vi "FPGA myRIOMain_v10.vi"() -> ()   [LabVIEW 2019]
doc: "Main FPGA VI\nUse the bitfile generated by this VI in the real-time code.\n\nv5: 16-pt Moving Average filter in AI sample loop"
uses:
  TypeDefs/AO mode TabCtrl.ctl
  TypeDefs/SamplingModeEnum_v2.ctl
  <vilib>/Platform/TimedLoop/XDataNode/timing_clust.ctl
  <vilib>/Platform/TimedLoop/XDataNode/nitl_modes.ctl
  <vilib>/Platform/TimedLoop/XDataNode/wakeup.ctl
  <vilib>/rvi/Emulation/niFpgaGetClockAttributes.vi
  <vilib>/rvi/Emulation/niFpgaSctlEmulationGetInTimedLoop.vi
  <vilib>/rvi/Emulation/niFpgaEmulationReportErrorSimple.vi
  <vilib>/rvi/eio/common/nirviEmuTemplateMethod_errors.vi
  <vilib>/rvi/Emulation/niFpgaEmulationIsFPGAContextNoSignature.vi
  <vilib>/rvi/errors/niFpgaSetErrorForExecOnDevCompSimple.vi
  <vilib>/rvi/eio/common/nirviEmuReportErrorAndStop.vi
  <vilib>/rvi/DataTransferAndStorage/Container/Common/niFpgaContainerGetUniqueNameForEmu.vi
  <vilib>/rvi/FIFO/Fifo_Resource/nirvififoEmulationSetSize.vi
  <vilib>/rvi/FIFO/Fifo_Resource/nirviFifoEmulationQueueMgr.vi
  <instcachedir>/0/nirviFifoEmulationQueueMgr_E5CAEC123FF24DC58D834DCA3CDAA9B5.lvgen/nirviFifoEmulationQueueMgr_E5CAEC123FF24DC58D834DCA3CDAA9B5_003.vi
  <vilib>/rvi/FIFO/Fifo_Resource/nirvififoEmulationDetermineInputValidOut.vi
  <vilib>/rvi/FIFO/Fifo_Resource/nirvififoEmulationCreateLock.vi
  <vilib>/rvi/Emulation/niFpgaProcessEmulError.vi
  <vilib>/rvi/FIFO/Fifo_Resource/nirvififoEmulationObtainLock.vi
  <vilib>/rvi/FIFO/Fifo_Resource/nirvififoEmulationReleaseLock.vi
  <vilib>/rvi/occurrence/nirviWaitOnOccurrenceBase.vi
  <vilib>/rvi/errors/nirviReportUnexpectedCaseInternalError.vi
  <vilib>/rvi/errors/nirviReportUnexpectedCaseInternalError (U32).vi
  <vilib>/rvi/Emulation/niFpgaCriticalErrorInLSC.vi
  <vilib>/Utility/error.llb/Clear Errors.vi
  <vilib>/rvi/Analysis/common/codeGenErrors/XNode/niFpgaXNodeCodeGenErrorHandle.vi
  <vilib>/eio/EIONode/EIONode.xnode
  <vilib>/rvi/DataTransferAndStorage/Container/XNode/niFpgaContainer.xnode
  <vilib>/rvi/FIFO/Fifo_Resource/nirvififoEmulationWrite.vi
  <vilib>/rvi/FIFO/Fifo_Resource/nirvififoEmulationRead.vi
  <vilib>/rvi/Analysis/measure/butterworth/XNode/niFpgaButterworthFilter.xnode
  <vilib>/rvi/FXPMathLib/FxpMul/XNode/nifxpmath_Multiplier.xnode
  <vilib>/rvi/Analysis/measure/LMRsmpl/XNode/niFPGA Rational Resampler.xnode
  <vilib>/Platform/TimedLoop/XDataNode/XDataNode.xnode
  FPGA functions/FPGA functions.lvlib
  <vilib>/Platform/TimedLoop/XDataNode/XDNodeRunTimeDep.lvlib
  <vilib>/rvi/FXPMathLib/sim/FxpSim.dll
panel:
  in  "scaled BW coefficients":i32[](array[numeric])=[-850883994, 1909449570, 3794062, -975456236, 2033039520, 4039635]
  in  "Sampling Mode":T1
  in  "AI Proc. Count [ticks]":u32
  in  "AI Count [ticks]":u32
  out "AI M Loop time [ticks]":u32
  out "FPGA AI DMA\nOverflow?":bool
  out "Sample Freq. \ntoo high?":bool
  out "Processing Loop time [ticks]":u32
  in  "AO mode":T2
  in  "AO Out [V]":fxp<+/-,18,5> format="%#.6g"
  in  "AO enable?":bool
  out "AI In [V]":fxp<+/-,24,5> format="%#.10g"
  out "FPGA AO DMA\nOverflow?":bool
  out "Int. Output":i16
  out "Raw Int. Input":fxp<+/-,22,12> format="%.8g"
  out "AO Loop time [ticks]":u32
  out "AI Loop time [ticks]":u32
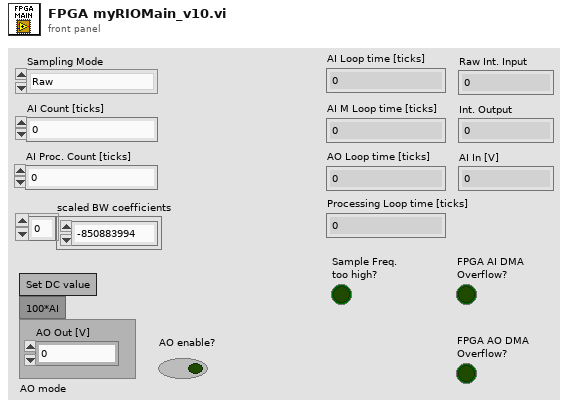
[diagram p1: front panel]
types:
  T1 = typedef "SamplingModeEnum_v2.ctl" = enum16{"Raw", "M64 - Resampling", "2nd-order Butterworth", "4th-order Butterworth", "64pt-MA", "128pt-MA", "256pt-MA"}
  T2 = typedef "AO mode TabCtrl.ctl" = enum32{"Set DC value", "100*AI"}
  T3 = typedef "XDNodeRunTimeDep.lvlib/timing_clust.ctl" = cluster{"Expected End [f-1]":u64, "Actual End [f-1]":u64, "Finished Late? [f-1]":bool, "Expected End [i-1]":u64, "Actual End [i-1]":u64, "Finished Late? [i-1]":bool, "Expected Start [i]":u64, "Actual Start [i]":u64, "Expected Start [f]":u64, "Actual Start [f]":u64, "Source Name":string, "Structure Name":string, "Period":i64, "Deadline":i64, "Offset":i64, "Start":i64, "Priority":i32, "Timeout":i32, "Mode":T4, "Wakeup Reason":T5, "Error":errorcluster, "Source Type":string, "Secondary Source Type":string, "Global End Time":u64, "Global Start Time":u64, "Frame Duration":u64, "Iteration Duration":u64, "Assigned CPU":i32, "I/O Scan Engine Mode":u32}
  T4 = typedef "XDNodeRunTimeDep.lvlib/nitl_modes.ctl" = enum32{"No Change", "Process missed periods, maintain original phase", "Discard missed periods, maintain original phase", "Process missed periods, ignore original phase", "Discard missed periods, ignore original phase"}
  T5 = typedef "XDNodeRunTimeDep.lvlib/wakeup.ctl" = enum32{"Normal", "Aborted", "Asynchronous wakeup", "Timing source error", "Timed loop error", "Timeout"}
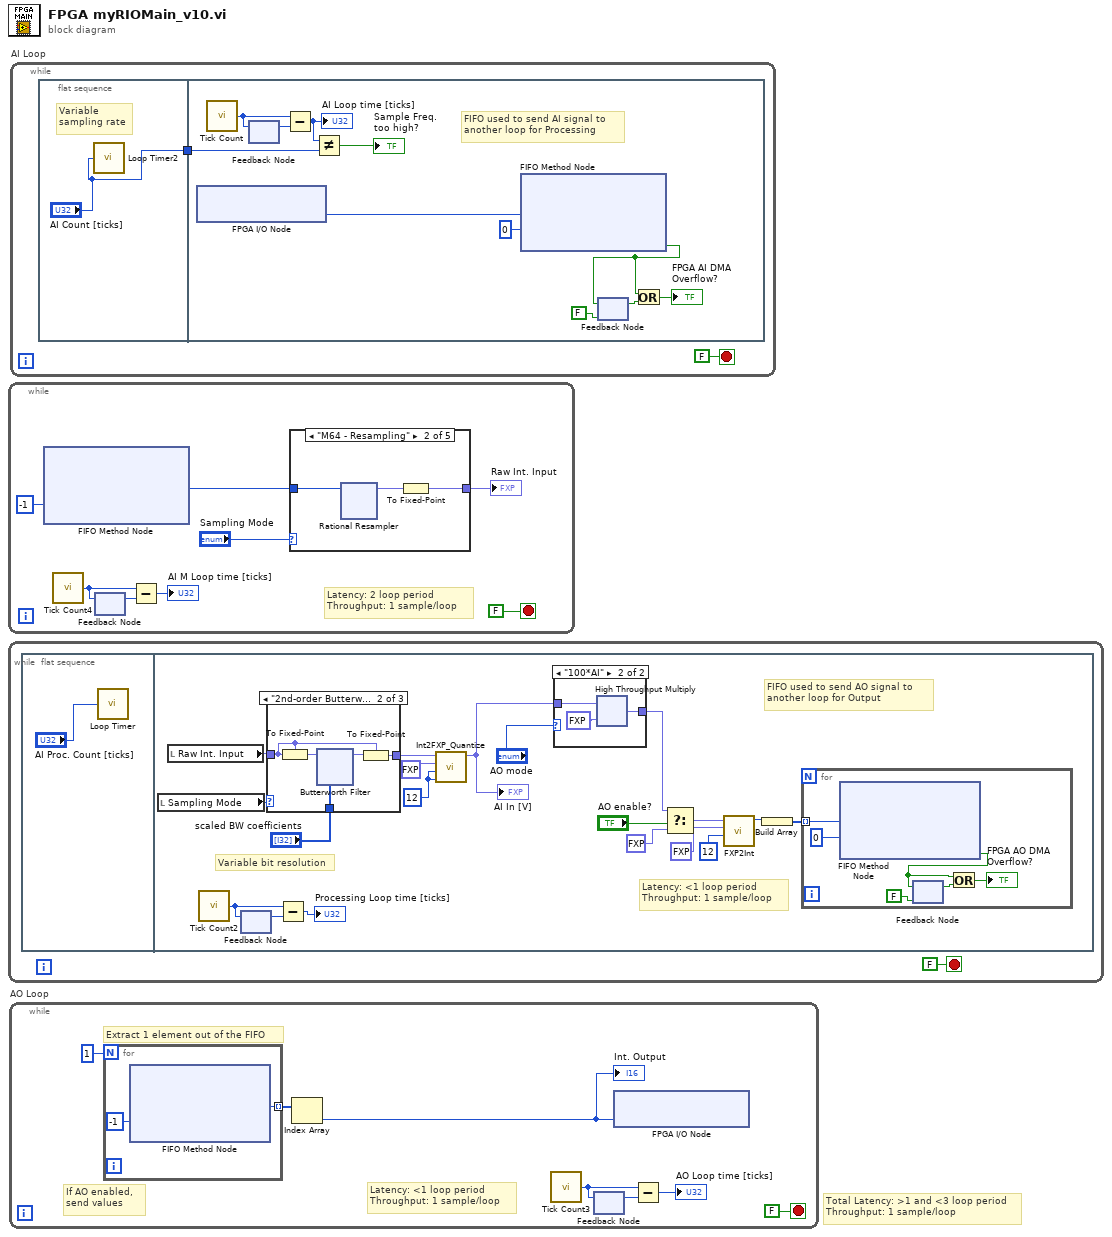
[diagram p0: block diagram]
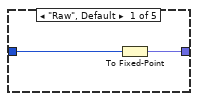
[diagram p2: hidden frame]
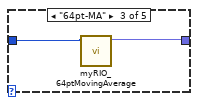
[diagram p3: hidden frame]
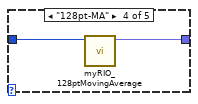
[diagram p4: hidden frame]
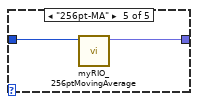
[diagram p5: hidden frame]
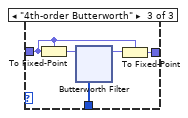
[diagram p7: hidden frame]
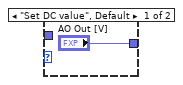
[diagram p8: hidden frame]
diagram:
  # "Total Latency: >1 and <3 loop period\nThroughput: 1 sample/loop"
  n1 = while {
    stop <- FALSE stop-if-true
    # "Latency: 2 loop period\nThroughput: 1 sample/loop"
    n2 = xnode ("FIFO Method Node")("Timeout"=-1) -> ("Element"=w1:i16)  [unwired: 1 in, 2 out]
    n3 = call "Tick Count4"() -> ("Tick Count(Ticks)"=w7:u32)
    n4 = feedback #1() -> (w6:u32)  [unwired: 1 in]
    n5 = feedback-in #1(w7) -> ()
    n6 = Subtract(x=w7, y=w6) -> (x-y=→"AI M Loop time [ticks]":u32)
    n7 = case shown="\"M64 - Resampling\"" "Sampling Mode" {
      tunnel: [w10 w11 w48 w50 w52] -> w3
      tunnel: w1 -> [w9 w13 w49 w51 w53]
      frame "Raw", Default {
        n8 = To Fixed-Point(number=w9) -> (fixed-point=w10:fxp<+/-,22,12>)  [unwired: 1 in]
      }
      frame "M64 - Resampling" {
        n9 = xnode "Rational Resampler"("input data"=w13) -> ("output data"=w12:fxp<+/-,18,16>)  [unwired: 2 out]
        n10 = To Fixed-Point(number=w12) -> (fixed-point=w11:fxp<+/-,22,12>)  [unwired: 1 in]
      }
      frame "64pt-MA" {
        n11 = call "myRIO_64ptMovingAverage.vi"("Raw input"=w49) -> ("Avg. output"=w48:fxp<+/-,22,12>)  [unwired: 10 in]
      }
      frame "128pt-MA" {
        n12 = call "myRIO_128ptMovingAverage.vi"("Raw input"=w51) -> ("Avg. output"=w50:fxp<+/-,22,12>)  [unwired: 10 in]
      }
      frame "256pt-MA" {
        n13 = call "myRIO_256ptMovingAverage.vi"("Raw input"=w53) -> ("Avg. output"=w52:fxp<+/-,22,12>)  [unwired: 10 in]
      }
    }
    "Raw Int. Input" <- w3
  }
  n14 = while {
    stop <- FALSE stop-if-true
    n15 = flat-sequence {
      frame #0 {
        n16 = call "Loop Timer"("Count(Ticks)"="AI Proc. Count [ticks]") -> ()  [unwired: 1 out]
      }
      frame #1 {
        w56 = i8 12 ("Input Bit resolution")
        # "Variable bit resolution"
        # "Latency: <1 loop period\nThroughput: 1 sample/loop"
        # "FIFO used to send AO signal to \nanother loop for Output"
        n17 = local read "Sampling Mode"() -> (w61:T1)
        n18 = local read "Raw Int. Input"() -> (w62:fxp<+/-,22,12>)
        n19 = call "Tick Count2"() -> ("Tick Count(Ticks)"=w65:u32)
        n20 = feedback #2() -> (w64:u32)  [unwired: 1 in]
        n21 = feedback-in #2(w65) -> ()
        n22 = case shown="\"2nd-order Butterworth\"" w61 {
          tunnel: [w75 w79 w92] -> w59
          tunnel: w62 -> [w75 w76 w89]
          tunnel: "scaled BW coefficients" -> [_ w77 w90]
          frame "Raw", Default {
          }
          frame "2nd-order Butterworth" {
            n23 = To Fixed-Point(fixed-point type=w76, number=w76) -> (fixed-point=w80:fxp<+/-,22,12>)
            n24 = xnode "Butterworth Filter"("input data"=w80, "scaled coefficients"=w77) -> ("output data"=w78:fxp<+/-,26,16>)  [unwired: 1 in]
            n25 = To Fixed-Point(fixed-point type=w76, number=w78) -> (fixed-point=w79:fxp<+/-,22,12>)
          }
          frame "4th-order Butterworth" {
            n26 = To Fixed-Point(fixed-point type=w89, number=w89) -> (fixed-point=w93:fxp<+/-,22,12>)
            n27 = xnode "Butterworth Filter"("input data"=w93, "scaled coefficients"=w90) -> ("output data"=w91:fxp<+/-,26,16>)  [unwired: 1 in]
            n28 = To Fixed-Point(fixed-point type=w89, number=w91) -> (fixed-point=w92:fxp<+/-,22,12>)
          }
        }
        n29 = Subtract(x=w65, y=w64) -> (x-y=→"Processing Loop time [ticks]":u32)
        n30 = call "Int2FXP_Quantize.vi"("Output Bit resolution"=w56, "Input Bit resolution"=w56, "Multiplier"=fxp<+,8,4> 10.0, "Input (Int)"=w59) -> ("Output (FXP)"=w58:fxp<+/-,24,5>)  [unwired: 7 in]
        "AI In [V]" <- w58
        n31 = case shown="\"100*AI\"" "AO mode" {
          tunnel: ["AO Out [V]" w103] -> w67
          tunnel: w58 -> [_ w105]
          frame "Set DC value", Default {
          }
          frame "100*AI" {
            n32 = xnode ("High Throughput Multiply")("x"=w105, "y"=fxp<+,5,7> 100.0) -> ("x*y"=w103:fxp<+/-,18,5>)
          }
        }
        n33 = Select(t=w67, s="AO enable?", f=fxp<+/-,18,5> 0.0) -> (s? t:f=w68:fxp<+/-,18,5>)
        n34 = call "FXP2Int.vi"("Output Bit resolution"=i8 12 ("Bit resolution"), "Multiplier"=fxp<+,18,-1> 0.10000038146972656, "Input (FXP)"=w68) -> ("Output (Int)"=w74:i16)  [unwired: 8 in]
        n35 = Build Array(w74) -> (w69:i16[])
        n36 = for {
          tunnel: w69 -> [w108] mode=indexing
          n37 = xnode ("FIFO Method Node")("Element"=w108, "Timeout"=0) -> ("Timed Out?"=w106:bool)  [unwired: 1 in, 1 out]
          n38 = feedback-in #3(w106) -> ()
          n39 = feedback #3(FALSE ("Timed Out?")) -> (w110:bool)
          n40 = Or(x=w106, y=w110) -> (x .or. y?=→"FPGA AO DMA\nOverflow?":bool)
        }
      }
    }
  }
  n41 = while "AO Loop" {
    stop <- FALSE stop-if-true
    # "Latency: <1 loop period\nThroughput: 1 sample/loop"
    # "If AO enabled, \nsend values"
    # "Extract 1 element out of the FIFO"
    n42 = for {
      N: 1 -> [_]
      tunnel: [w120] -> w114 mode=indexing
      n43 = xnode ("FIFO Method Node")("Timeout"=-1) -> ("Element"=w120:i16)  [unwired: 1 in, 2 out]
    }
    n44 = Index Array(array=w114) -> (element=w112:i16)  [unwired: 1 in]
    "Int. Output" <- w112
    n45 = call "Tick Count3"() -> ("Tick Count(Ticks)"=w117:u32)
    n46 = feedback #4() -> (w116:u32)  [unwired: 1 in]
    n47 = feedback-in #4(w117) -> ()
    n48 = xnode "FPGA I/O Node"("ConnectorC/AO0"=w112) -> ()  [unwired: 1 in, 1 out]
    n49 = Subtract(x=w117, y=w116) -> (x-y=→"AO Loop time [ticks]":u32)
  }
  n50 = while "AI Loop" {
    stop <- FALSE stop-if-true
    n51 = flat-sequence {
      tunnel: ["AI Count [ticks]"] -> w121
      tunnel: w121 -> [w131]
      frame #0 {
        # "Variable\nsampling rate"
        n52 = call "Loop Timer2"("Count(Ticks)"="AI Count [ticks]") -> ()  [unwired: 1 out]
      }
      frame #1 {
        # "FIFO used to send AI signal to \nanother loop for Processing"
        n53 = xnode "FPGA I/O Node"() -> ("ConnectorC/AI0"=w124:i16)  [unwired: 1 in, 1 out]
        n54 = call "Tick Count"() -> ("Tick Count(Ticks)"=w134:u32)
        n55 = feedback #5() -> (w133:u32)  [unwired: 1 in]
        n56 = feedback-in #5(w134) -> ()
        n57 = Subtract(x=w134, y=w133) -> (x-y=w132:u32)
        "AI Loop time [ticks]" <- w132
        n58 = Not Equal?(x=w132, y=w131) -> (x != y?=→"Sample Freq. \ntoo high?":bool)
        n59 = xnode ("FIFO Method Node")("Element"=w124, "Timeout"=0) -> ("Timed Out?"=w125:bool)  [unwired: 1 in, 1 out]
        n60 = feedback #6(FALSE ("Timed Out?")) -> (w127:bool)
        n61 = feedback-in #6(w125) -> ()
        n62 = Or(x=w125, y=w127) -> (x .or. y?=→"FPGA AI DMA\nOverflow?":bool)
      }
    }
  }
